vi "CRYGet Frame and Graph VIRef.vi"(10 "Panel Idx":i32, 11 "Graph VIRef Array":T1(array[cluster])) -> (0 "Icon Ring":i32, 1 "Graph VIRef":refnum<vi>, 2 "Frame VIRef":refnum<vi>, 3 "Graph VIRef Array Index":i32=-1, 4 "Graph Type":string)   [LabVIEW 2013]
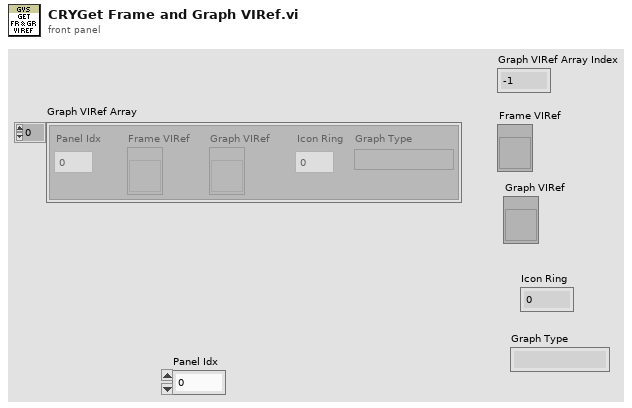
[diagram p1: front panel]
types:
  T1 = cluster{"Graph VIRef":refnum<vi>, "Panel Idx":i32, "Frame VIRef":refnum<vi>, "Icon Ring":i32, "Graph Type":string}[]
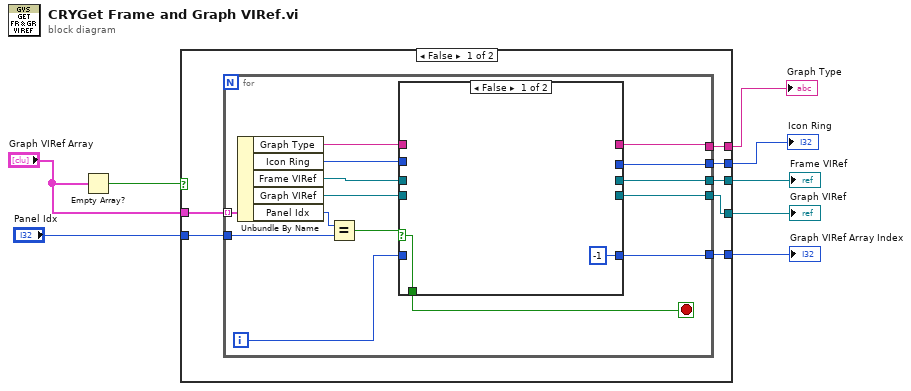
[diagram p0: block diagram]
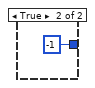
[diagram p3: hidden frame]
diagram:
  n1 = Empty Array?(array="Graph VIRef Array") -> (empty?=w1:bool)
  n2 = case shown="False" w1 {
    tunnel: "Panel Idx" -> [w15 _]
    tunnel: [w14 -1] -> w7
    tunnel: [w13 _] -> w6
    tunnel: [w12 _] -> w5
    tunnel: [w11 _] -> w4
    tunnel: [w10 _] -> w3
    tunnel: "Graph VIRef Array" -> [w9 _]
    frame False {
      n3 = for {
        tunnel: w9 -> [w30] mode=indexing
        tunnel: w15 -> [w28]
        tunnel: [w23] -> w13
        tunnel: [w22] -> w12
        tunnel: [w20] -> w14
        tunnel: [w18] -> w11
        tunnel: [w16] -> w10
        i -> [w21]
        stop <- w26 stop-if-true
        n4 = Unbundle By Name(w30) -> ("Graph Type"=w17:string, "Icon Ring"=w19:i32, "Frame VIRef"=w25:refnum<vi>, "Graph VIRef"=w24:refnum<vi>, "Panel Idx"=w29:i32)
        n5 = Equal?(x=w29, y=w28) -> (x = y?=w27:bool)
        n6 = case shown="False" w27 {
          selector: w27 -> [w32 w38]
          tunnel: [w32 w38] -> w26
          tunnel: w25 -> [_ w37]
          tunnel: w24 -> [_ w36]
          tunnel: [_ w37] -> w23
          tunnel: [_ w36] -> w22
          tunnel: w21 -> [_ w35]
          tunnel: [-1 w35] -> w20
          tunnel: [_ w34] -> w18
          tunnel: w19 -> [_ w34]
          tunnel: w17 -> [_ w33]
          tunnel: [_ w33] -> w16
          frame False {
          }
          frame True {
          }
        }
      }
    }
    frame True {
    }
  }
  "Graph VIRef Array Index" <- w7
  "Frame VIRef" <- w6
  "Graph VIRef" <- w5
  "Icon Ring" <- w4
  "Graph Type" <- w3
